vi "Write Generate Report Msg.vi"(10 "User Interface.lvlib:Generate Report Msg.lvclass":refnum<class "Generate Report Msg.lvclass">, 11 "User Interface in":refnum<class "User Interface.lvclass">) -> (3 "User Interface out":refnum<class "User Interface.lvclass">)   [LabVIEW 2017, in "User Interface.lvlib" / "User Interface.lvclass"]
uses:
  User Interface.lvclass
  User Interface Messages/Generate Report Msg/Generate Report Msg.lvclass
  User Interface.lvclass/User Interface.ctl
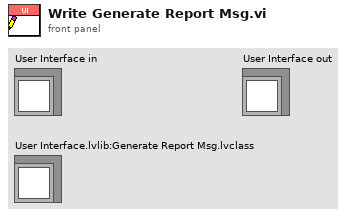
[diagram p1: front panel]
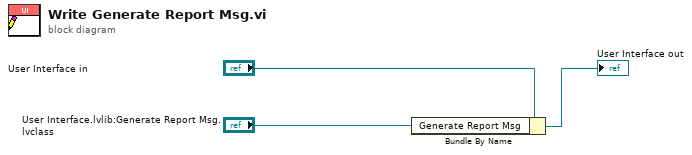
[diagram p0: block diagram]
diagram:
  n1 = Bundle By Name(cluster="User Interface in", "Generate Report Msg"="User Interface.lvlib:Generate Report Msg.lvclass") -> (→"User Interface out":refnum<class "User Interface.lvclass">)
